vi "Dashboard Main.vi"() -> ()   [LabVIEW 2012]
uses:
  2012/code/Dashboard/High Priority Dash Data.ctl
  Control 3.ctl
  Control 4.ctl
  Control 2.ctl
  Control 5.ctl
  <vilib>/event_ctls.llb/eventvkey.ctl
  high priority dash data.vi
  low priority dash data.vi
  <vilib>/Utility/config.llb/Read Key (String).vi
  <vilib>/Utility/config.llb/Read Key (I32).vi
  <vilib>/Utility/config.llb/Write Key (String).vi
  <vilib>/Utility/config.llb/Write Key (I32).vi
  <vilib>/Utility/config.llb/NI_LVConfig.lvlib
panel:
  out "Battery Value":dbl(slide) scale=0.0..14.0 scale format="%#_2e"
  out "Battery":sgl(graph)
  in  "Camera Settings":T1={"Frate Rate"=30, "Compression"=30, "Size"=1} {"Frate Rate" scale=1.0..30.0; "Size" items=["640x480", "320x240", "160x120"]}
  out "Mode":T2(ring)=enum."Auto Disabled"
  out "Camera IP":string
  out "JS1 Z":dbl(slide) scale=-1.0..1.0 scale format="%#_2e"
  out "JS2 Z":dbl(slide) scale=-1.0..1.0 scale format="%#_2e"
  out "Joystick 1":cluster{"X":dbl, "Y":dbl}[](graph)
  out "Joystick 2":cluster{"X":dbl, "Y":dbl}[](graph)
  out "JS Buttons 1":T3
  out "JS Buttons 2":T3
  out "MotorSlide4":dbl(slide) scale=-1.0..1.0 scale format="%#_2e"
  out "MotorSlide3":dbl(slide) scale=-1.0..1.0 scale format="%#_2e"
  out "MotorSlide2":dbl(slide) scale=-1.0..1.0 scale format="%#_2e"
  in  "MotorName3":string="Front Left"
  in  "MotorName4":string="Front Right"
  in  "MotorName1":string="Rear Left"
  in  "MotorName2":string="Rear Right"
  out "MotorChart4":dbl(graph)
  out "MotorChart3":dbl(graph)
  out "MotorChart2":dbl(graph)
  out "MotorSlide1":dbl(slide) scale=-1.0..1.0 scale format="%#_2e"
  out "MotorChart1":dbl(graph)
  out "Robot IP":string
  in  "Dashboard Tab":enum32{"Operation", "Test", "Checklist"}(tab)
  out "XY Graph":cluster{"Y":dbl[], "Y":dbl[]}[](graph)
  in  "Slider":dbl(slide) scale=0.0..100.0 scale format="%#_3g"
  in  "On/Off":bool caption="Solenoid"
  in  "Test Name":u16(ring) items=["Select the test to run..."]
  in  "Test Tree":string(tree)
  in  "Motor":cluster{"Value":dbl, "Enable":bool} {"Value" scale=-1.0..1.0 scale format="%#_3g"}
  out "Progress":T4 {"Test Progress" scale=0.0..100.0}
  in  "Rev/Fwd":cluster{"Forward":bool, "Reverse":bool}
  in  "Ring":u16(ring) items=["Auto", "Fixed indoor", "Fixed outdoor 1", "Fixed outdoor 2", "Fixed fluorescent 1", "Fixed fluorescent 2", "Hold current"]
  in  "Listbox":i32(listbox)
  in  "Viewer":T5(tab)
  out "Mbps":dbl format="%#.1g"
  in  "Enable":bool
  in  "DB Camera Config":bool
  out "Mbps":bool
  out "fps":dbl format="%#.1g"
  out "Image Error Message":string="Timeout in Camera Communications"
  out "Camera Image":T6(plugin-control)
  out "Buttons 1":cluster{"1":bool, "2":bool, "3":bool}
  out "Kinect 1":cluster{"X":dbl, "Y":dbl, "Z":dbl} {"X" scale=1.0..-1.0; "Y" scale=1.0..-1.0; "Z" scale=1.0..-1.0}
  out "Buttons 2":cluster{"1":bool, "2":bool, "3":bool}
  out "Kinect 2":cluster{"X":dbl, "Y":dbl, "Z":dbl} {"X" scale=1.0..-1.0; "Y" scale=1.0..-1.0; "Z" scale=1.0..-1.0}
  out "Version":string
  out "Skeleton Picture":picture
  out "Players":i8
  out "Tree":string(tree)
  # "Drive & Motors"
  # "Robot IP:"
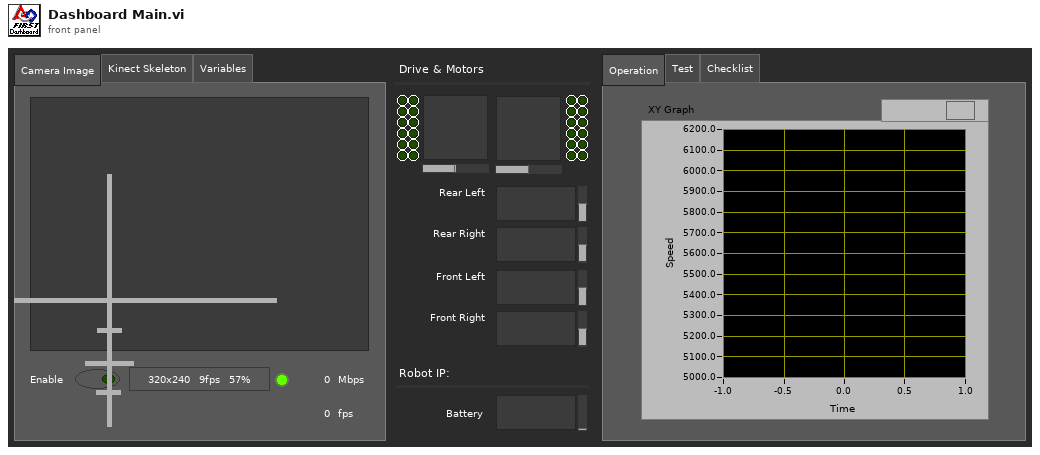
[diagram p1: front panel]
types:
  T1 = cluster{"Frate Rate":i32, "Compression":i32, "Size":u16}
  T2 = enum8{"Tele-Op Disabled", "Tele-Op Enabled", "Auto Disabled", "Auto Enabled", "Test Disabled", "Test Enabled", ""}
  T3 = cluster{bool, bool, bool, bool, bool, bool, bool, bool, bool, bool, bool, bool}
  T4 = cluster{"Test Progress":u8, "Test Progress Text":string}
  T5 = enum32{"Camera Image", "Kinect Skeleton", "Variables"}
  T6 = typedef "IMAQ Image.ctl" = refnum<image>
  T7 = typedef "Control 4.ctl" = cluster{"shooter speed":dbl}
  T8 = typedef "Control 3.ctl" = cluster{"shooter speed":dbl}
  T9 = typedef "High Priority Dash Data.ctl" = cluster{cluster{bool, i32, i32, i32, i32}, cluster{bool, i32, i32, i32, i32}, cluster{bool, i32, i32, i32, i32}, cluster{bool, i32, i32, i32, i32}}
  T10 = typedef "Image Type" = u32
  T11 = typedef "LVBoundsTypeDef.ctl" = cluster{"Width":u32, "Height":u32}
  T12 = typedef "SkeletonTrackState.ctl" = enum32{"NotTracked", "PositionOnly", "Tracked"}
  T13 = cluster{"TrackingState":u8[], "Position":cluster{"x":sgl, "y":sgl, "z":sgl}, cluster{"x":sgl, "y":sgl, "z":sgl, sgl}[], "TrackState":T12}
  T14 = cluster{cluster{"ScaledToPercentRange":dbl, "ScaledToPercentRange":dbl, "ScaledToPercentRange":dbl}, cluster{bool, bool, bool}}[]
  T15 = cluster{cluster{"ScaledToPercentRange":dbl, "ScaledToPercentRange":dbl, "ScaledToPercentRange":dbl}, cluster{bool, bool, bool}}
  T16 = cluster{"ScaledToPercentRange":dbl, "ScaledToPercentRange":dbl, "ScaledToPercentRange":dbl}
  T17 = typedef "LVRectTypeDef.ctl" = cluster{"Left":i16, "Top":i16, "Right":i16, "Bottom":i16}
  T18 = typedef "Control 5.ctl" = cluster{dbl}
  T19 = typedef "Control 2.ctl" = cluster{"shooter speed":dbl}
  T20 = cluster{"Competition mode":bool, "Robot Link":bool, "Autonomous":bool, "Enabled":bool, "E-Stop":bool, "Simulated":bool, "TestMode":bool, "Docked Window":bool}
  T21 = cluster{"Boolean Array[0]":bool, "Boolean Array[1]":bool, "Boolean Array[2]":bool, "Boolean Array[3]":bool, "Boolean Array[4]":bool, "Boolean Array[5]":bool, "Boolean Array[6]":bool, "Boolean Array[7]":bool, "Boolean Array[8]":bool, "Boolean Array[9]":bool, "Boolean Array[10]":bool, "Boolean Array[11]":bool}
  T22 = typedef "NI_LVConfig.lvlib/Config Data RefNum.ctl" = refnum<k1>
  T23 = typedef "eventvkey.ctl" = enum16{"ASCII", "Enter", "Return", "Shift", "Ctrl", "Alt", "Cmd", "Opt", "Caps", "NumLock", "Clear", "Break", "Up", "Down", "Left", "Right", "Insert", "Delete", "Home", "End", "PageUp", "PageDown", "Escape", "Help", "Pause", "ScrollLock", "F1", "F2", "F3", "F4", "F5", "F6", "F7", "F8", "F9", "F10", "F11", "F12", "F13", "F14", "F15", "F16", "F17", "F18", "F19", "F20", "F21", "F22", "F23", "F24", "Play", "VolumeUp", "VolumeDown", "Mute", "Two Byte Char"}
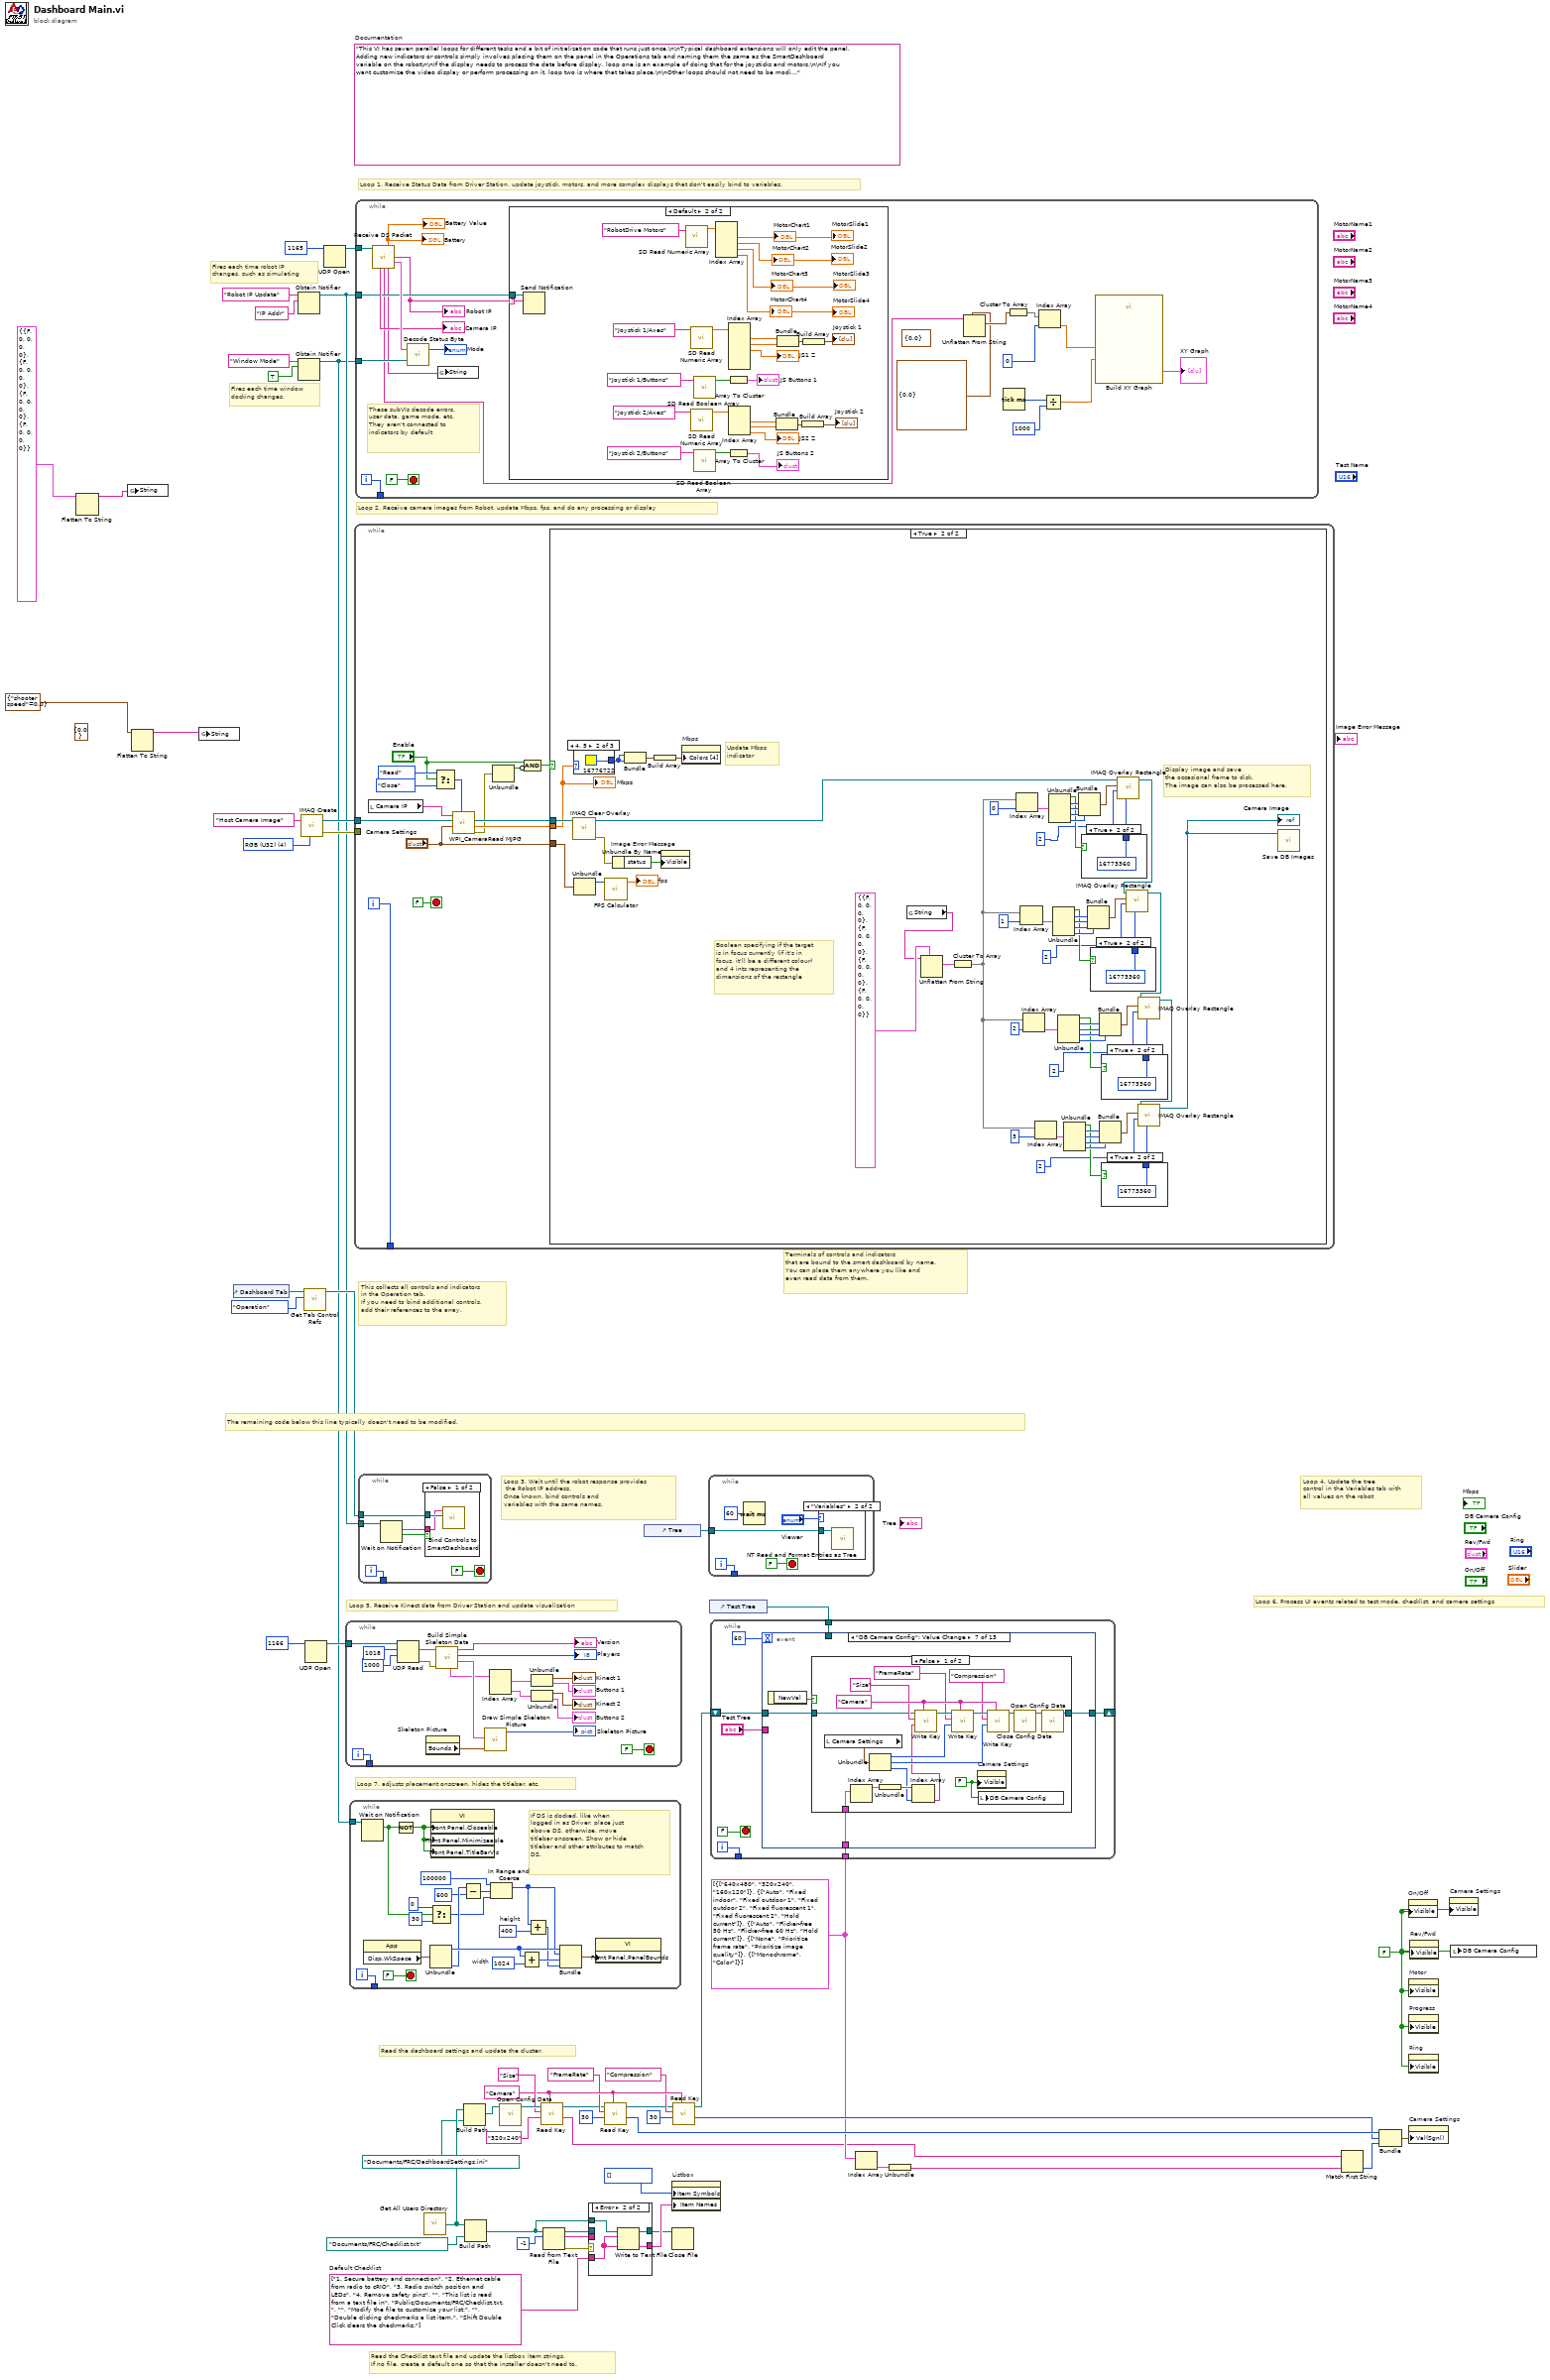
[diagram p0: block diagram]
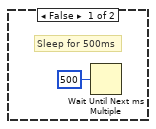
[diagram p3: hidden frame]
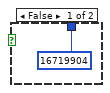
[diagram p4: hidden frame]
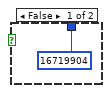
[diagram p5: hidden frame]
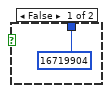
[diagram p6: hidden frame]
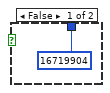
[diagram p7: hidden frame]
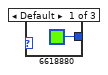
[diagram p8: hidden frame]
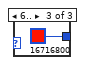
[diagram p9: hidden frame]
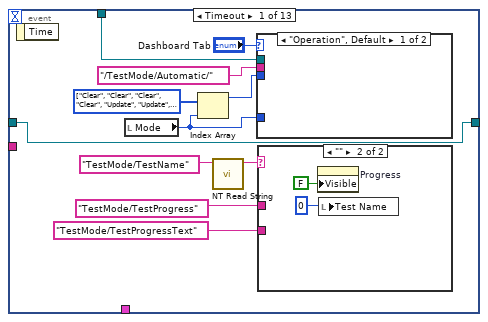
[diagram p11: hidden frame]
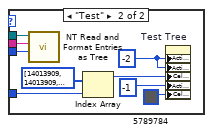
[diagram p12: hidden frame]
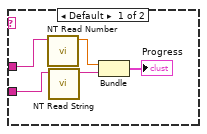
[diagram p13: hidden frame]
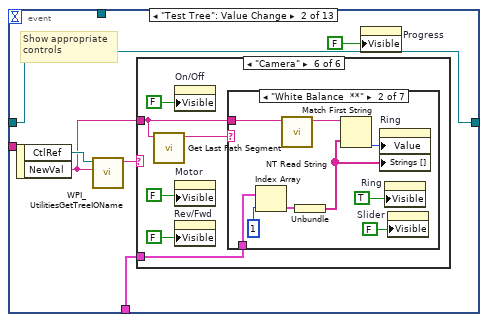
[diagram p14: hidden frame]
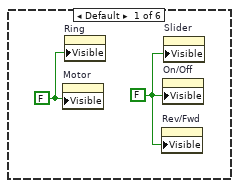
[diagram p15: hidden frame]
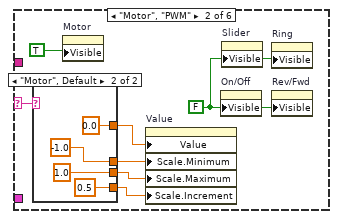
[diagram p16: hidden frame]
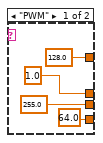
[diagram p17: hidden frame]
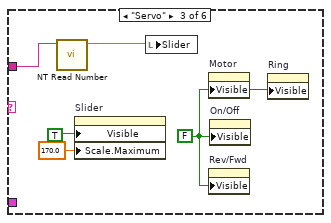
[diagram p18: hidden frame]
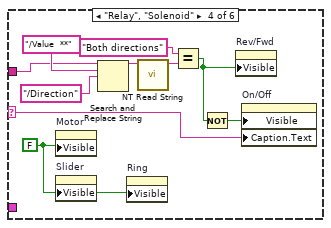
[diagram p19: hidden frame]
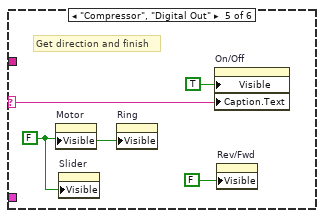
[diagram p20: hidden frame]
diagram:
  (unwired) T8 {"shooter speed"=0.0} ("Cluster")
  w25 = "Camera"
  w17 = cluster{string[]}[] [{["640x480", "320x240", "160x120"]}, {["Auto", "Fixed indoor", "Fixed outdoor 1", "Fixed outdoor 2", "Fixed fluorescent 1", "Fixed fluorescent 2", "Hold current"]}, {["Auto", "Flicker-free 50 Hz", "Flicker-free 60 Hz", "Hold current"]}, {["None", "Prioritize frame rate", "Prioritize image quality"]}, {["Monochrome", "Color"]}]
  w33 = string[] ["1. Secure battery and connection", "2. Ethernet cable from radio to cRIO", "3. Radio switch position and LEDs", "4. Remove safety pins", "", "This list is read from a text file in", "Public/Documents/FRC/Checklist.txt.", "", "Modify the file to customize your list.", "", "Double clicking checkmarks a list item.", "Shift Double Click clears the checkmarks."]  # Default Checklist
  w31 = FALSE ("Visible")
  (unwired) "This VI has seven parallel loops for different tasks and a bit of initialization code that runs just once.\n\nTypical dashboard extensions will only edit the panel. Adding new indicators or controls simply involves placing them on the panel in the Operations tab and naming them the same as the SmartDashboard variable on the robot\n\nIf the display needs to process the data before display, loop one is an example of doing that for the joysticks and motors.\n\nIf you want customize the video display or perform processing on it, loop two is where that takes place.\n\nOther loops should not need to be modified. They are pretty standard, and document the task they perform."  # Documentation
  w54 = T10 4 items=["Grayscale (U8)", "Grayscale (I16)", "Grayscale (SGL)", "Complex (CSG)", "RGB (U32)", "HSL (U32)", "RGB (U64)"] ("Image Type")
  # "Fires each time robot IP\nchanges, such as simulating"
  # "Fires each time window\ndocking changes."
  # "Read the Checklist text file and update the listbox item strings.\nIf no file, create a default one so that the installer doesn't need to."
  # "This collects all controls and indicators\nin the Operation tab.\nIf you need to bind additional controls,\nadd their references to the array."
  # "The remaining code below this line typically doesn't need to be modified."
  # "Loop 6. Process UI events related to test mode, checklist, and camera settings"
  # "Read the dashboard settings and update the cluster."
  # "Terminals of controls and indicators\nthat are bound to the smart dashboard by name.\nYou can place them anywhere you like and\neven read data from them."
  # "Loop 4. Update the tree\ncontrol in the Variables tab with\nall values on the robot"
  # "Loop 3. Wait until the robot response provides\n the Robot IP address.\nOnce known, bind controls and\nvariables with the same names."
  # "Loop 5. Receive Kinect data from Driver Station and update visualization"
  # "Loop 7. adjusts placement onscreen, hides the titlebar, etc."
  # "Loop 1. Receive Status Data from Driver Station, update joystick, motors, and more complex displays that don't easily bind to variables."
  # "Loop 2. Receive camera images from Robot, update Mbps, fps, and do any processing or display"
  n1 = Flatten To String(anything=T9 {{FALSE, 0, 0, 0, 0}, {FALSE, 0, 0, 0, 0}, {FALSE, 0, 0, 0, 0}, {FALSE, 0, 0, 0, 0}}) -> (data string=w3:string)  [unwired: 3 in, 2 out]
  n2 = global write "high priority dash data.vi" "String"(w3) -> ()
  n3 = Flatten To String(anything=T7 {"shooter speed"=0.0} ("Cluster")) -> (data string=w2:string)  [unwired: 3 in, 2 out]
  n4 = global write "low priority dash data.vi" "String"(w2) -> ()
  n5 = control-ref of="Dashboard Tab"() -> (w47:refnum<vi>)
  n6 = Obtain Notifier(name (unnamed)="Robot IP Update", notification data type="IP Addr" ("name (unnamed)")) -> (notifier out=w44:refnum<notifier>)  [unwired: 2 in, 2 out]
  n7 = Obtain Notifier(name (unnamed)="Window Mode", notification data type=TRUE) -> (notifier out=w37:refnum<notifier>)  [unwired: 2 in, 2 out]
  n8 = call "IMAQ Create"("Image Name"="Host Camera Image", "Image Type"=w54) -> ("New Image"=w52:T6, "error out"=w51:errorcluster)  [unwired: 2 in, 1 out]
  n9 = call <vilib>:"Get Tab Control Refs.vi"("Page Index"=enum32{"Operation", "Test"}."Operation" ("Dashboard Tab"), "TabControl in"=w47) -> ("ControlsOnPage"=w48:refnum<vi>[])  [unwired: 9 in]
  n10 = UDP Open(11:u16 1166 ("port")) -> (port=w49:refnum<k16>)  [unwired: 2 in, 4 out]
  n11 = UDP Open(11:u16 1165 ("port")) -> (port=w55:refnum<k16>)  [unwired: 2 in, 4 out]
  n12 = while {
    tunnel: w49 -> [w73]
    tunnel: [w58] -> _
    i -> [w58]
    stop <- FALSE stop-if-true
    n13 = UDP Read(connection ID=w73, max size (548)=1018 ("bytes to read"), timeout ms (25000)=1000) -> (data out=w67:string, error out=w57:errorcluster)  [unwired: 1 in, 3 out]
    n14 = property on="Skeleton Picture" class="Pict"() -> ("Bounds"=w69:T11)  [unwired: 2 in, 2 out]
    n15 = call "Build Simple Skeleton Data.vi"("error in (no error)"=w57, "data in"=w67) -> ("Skeleton Data"=w68:T13, "NumPlayers"=→"Players":i8, "Version String"=→"Version":string, "Simple Joystick Info"=w65:T14)  [unwired: 5 in, 1 out]
    n16 = call "Draw Simple Skeleton Picture.vi"("Bounds"=w69, "Simple Skeleton"=w68) -> ("new picture out"=→"Skeleton Picture":picture)  [unwired: 9 in]
    n17 = Index Array(array=w65) -> (element #1=w64:T15, element #2=w63:T15)  [unwired: 2 in]
    n18 = Unbundle(w64) -> (→"Kinect 1":T16, →"Buttons 1":cluster{bool, bool, bool})
    n19 = Unbundle(w63) -> (→"Kinect 2":T16, →"Buttons 2":cluster{bool, bool, bool})
  }
  n20 = while {
    tunnel: w37 -> [w94]
    tunnel: [w92] -> _
    i -> [w92]
    stop <- FALSE stop-if-true
    w84 = 1024  # width
    w87 = 400  # height
    # "If DS is docked, like when\nlogged in as Driver, place just\nabove DS, otherwise, move\ntitlebar onscreen. Show or hide\ntitlebar and other attributes to match\nDS."
    n21 = Wait on Notification(notifier=w94) -> (notification=w79:bool)  [unwired: 3 in, 3 out]
    n22 = property class="App"() -> ("Disp.WkSpace"=w90:T17)  [unwired: 2 in, 2 out]
    n23 = Not(x=w79) -> (.not. x?=w93:bool)
    n24 = Unbundle(w90) -> ("Left"=w88:i16, "Bottom"=w85:i16)  [unwired: 2 out]
    n25 = Select(t=0, s=w79, f=30) -> (s? t:f=w78:i32)
    n26 = property class="VI"("Front Panel.Closeable"=w93, "Front Panel.Minimizeable"=w93, "Front Panel.TitleBarVis"=w93) -> ()  [unwired: 2 in, 2 out]
    n27 = Subtract(x=w85, y=600) -> (x-y=w82:i32)
    n28 = In Range and Coerce(upper limit=100000, x=w82, lower limit=w78) -> (coerced(x)=w76:i32)  [unwired: 1 out]
    n29 = Add(x=w88, y=w84) -> (x+y=w89:i32)
    n30 = Add(x=w76, y=w87) -> (x+y=w86:i32)
    n31 = Bundle("Left"=w88, w76, w89, w86) -> (w91:cluster{"Left":i16, i32, i32, i32})  [unwired: 1 out]
    n32 = property class="VI"("Front Panel.PanelBounds"=w91) -> ()  [unwired: 2 in, 2 out]
  }
  n33 = while {
    tunnel: w52 -> [w105]
    tunnel: w51 -> [_]
    tunnel: [w108] -> _
    i -> [w108]
    stop <- FALSE stop-if-true
    n34 = local read "Camera IP"() -> (w107:string)
    n35 = Select(t=enum16{"Read", "Reopen", "Close"}."Read" ("Operation"), s="Enable", f=enum16{"Read", "Reopen", "Close"}."Close" ("Operation")) -> (s? t:f=w100:enum16{"Read", "Reopen", "Close"})
    n36 = call <vilib>:"WPI_CameraRead MJPG.vi"("Operation"=w100, "Camera Settings"="Camera Settings", "Image"=w105, "address"=w107) -> ("error out"=w99:errorcluster, "Bandwidth (kbps)"=w103:dbl, "Image Out"=w104:T6)  [unwired: 5 in]
    n37 = Unbundle(w99) -> ("status"=w97:bool)  [unwired: 2 out]
    n38 = Compound Arithmetic op=AND("Enable", invert w97) -> (w96:bool)
    n39 = case shown="True" w96 {
      tunnel: "Camera Settings" -> [_ w161]
      tunnel: w104 -> [_ w164]
      tunnel: w103 -> [_ w163]
      frame False {
        # "Sleep for 500ms"
        n40 = Wait Until Next ms Multiple(millisecond multiple=u32 500) -> ()  [unwired: 1 out]
      }
      frame True {
        # "Boolean specifying if the target\nis in focus currently (if it's in \nfocus, it'll be a different colour)\nand 4 ints representing the\ndimensions of the rectangle"
        # "Display image and save\nthe occasional frame to disk.\nThe image can also be processed here."
        # "Update Mbps\nindicator"
        n41 = call "IMAQ Clear Overlay"("Image"=w164) -> ("error out"=w168:errorcluster, "Image Out"=w113:T6)  [unwired: 2 in, 7 out]
        n42 = case shown="4, 5" w163 {
          tunnel: [u32 6618880 ("Color Box") u32 16776722 ("Color Box") u32 16716800 ("Color Box")] -> w165
          frame Default {
          }
          frame 4, 5 {
          }
          frame 6.. {
          }
        }
        n43 = Unbundle(w161) -> ("Frate Rate"=w160:i32)  [unwired: 2 out]
        n44 = call "FPS Calculator.vi"("Average Count"=w160) -> ("fps"=→"fps":dbl)  [unwired: 10 in]
        n45 = Unbundle By Name(w168) -> ("status"=w169:bool)
        n46 = Bundle("Color Box"=w165, "Color Box"=w165) -> (w167:cluster{"Color Box":u32, "Color Box":u32})  [unwired: 1 out]
        n47 = Build Array(w167) -> (w166:cluster{"Color Box":u32, "Color Box":u32}[])
        n48 = property on="Image Error Message" class="Str"("Visible"=w169) -> ()  [unwired: 2 in, 2 out]
        n49 = property on="Mbps" class="Bool (strict)"("Colors [4]"=w166) -> ()  [unwired: 2 in, 2 out]
        n50 = global read "high priority dash data.vi" "String"() -> (w114:string)
        n51 = Unflatten From String(type=T9 {{FALSE, 0, 0, 0, 0}, {FALSE, 0, 0, 0, 0}, {FALSE, 0, 0, 0, 0}, {FALSE, 0, 0, 0, 0}}, binary string=w114) -> (value=w151:T9)  [unwired: 1 in, 4 out]
        n52 = Cluster To Array(cluster=w151) -> (array=w111:cluster{bool, i32, i32, i32, i32}[])
        n53 = Index Array(array=w111, index=0) -> (element=w149:cluster{bool, i32, i32, i32, i32})
        n54 = Index Array(array=w111, index=1) -> (element=w140:cluster{bool, i32, i32, i32, i32})
        n55 = Index Array(array=w111, index=2) -> (element=w131:cluster{bool, i32, i32, i32, i32})
        n56 = Index Array(array=w111, index=3) -> (element=w122:cluster{bool, i32, i32, i32, i32})
        n57 = Unbundle(w149) -> (w152:bool, w153:i32, w154:i32, w156:i32, w155:i32)
        n58 = Unbundle(w140) -> (w142:bool, w143:i32, w144:i32, w146:i32, w145:i32)
        n59 = Unbundle(w131) -> (w133:bool, w134:i32, w135:i32, w137:i32, w136:i32)
        n60 = Unbundle(w122) -> (w124:bool, w125:i32, w126:i32, w128:i32, w127:i32)
        n61 = Bundle(w153, w154, w156, w155) -> (w158:cluster{i32, i32, i32, i32})  [unwired: 1 in]
        n62 = case shown="True" w152 {
          tunnel: [16719904 16773360] -> w157
          frame False {
          }
          frame True {
          }
        }
        n63 = Bundle(w143, w144, w146, w145) -> (w148:cluster{i32, i32, i32, i32})  [unwired: 1 in]
        n64 = case shown="True" w142 {
          tunnel: [16719904 16773360] -> w147
          frame False {
          }
          frame True {
          }
        }
        n65 = Bundle(w134, w135, w137, w136) -> (w139:cluster{i32, i32, i32, i32})  [unwired: 1 in]
        n66 = Bundle(w125, w126, w128, w127) -> (w130:cluster{i32, i32, i32, i32})  [unwired: 1 in]
        n67 = case shown="True" w133 {
          tunnel: [16719904 16773360] -> w138
          frame False {
          }
          frame True {
          }
        }
        n68 = case shown="True" w124 {
          tunnel: [16719904 16773360] -> w129
          frame False {
          }
          frame True {
          }
        }
        n69 = call "IMAQ Overlay Rectangle"("Color"=w157, "Drawing Mode (Frame)"=2, "Rectangle"=w158, "Image"=w113) -> ("Image Out"=w121:T6)  [unwired: 6 in, 1 out]
        n70 = call "IMAQ Overlay Rectangle"("Color"=w147, "Drawing Mode (Frame)"=2, "Rectangle"=w148, "Image"=w121) -> ("Image Out"=w120:T6)  [unwired: 6 in, 1 out]
        n71 = call "IMAQ Overlay Rectangle"("Color"=w138, "Drawing Mode (Frame)"=2, "Rectangle"=w139, "Image"=w120) -> ("Image Out"=w119:T6)  [unwired: 6 in, 1 out]
        n72 = call "IMAQ Overlay Rectangle"("Color"=w129, "Drawing Mode (Frame)"=2, "Rectangle"=w130, "Image"=w119) -> ("Image Out"=w112:T6)  [unwired: 6 in, 1 out]
        "Camera Image" <- w112
        n73 = call "Save DB Images.vi"("Image"=w112) -> ()  [unwired: 2 in, 1 out]
        "Mbps" <- w163
      }
    }
  }
  n74 = while {
    tunnel: w55 -> [w199]
    tunnel: w44 -> [w193]
    tunnel: w37 -> [w197]
    tunnel: [w194] -> _
    i -> [w194]
    stop <- FALSE stop-if-true
    (unwired) T19 {"shooter speed"=0.0} ("Cluster")
    # "These subVIs decode errors, user data, game mode, etc.\nThey aren't connected to indicators by default"
    n75 = call "Receive DS Packet.vi"("Recv Socket"=w199) -> ("Battery"=→"Battery" →"Battery Value":sgl, "Robot IP Address"=w192:string, "Status"=w200:T20, "Camera IP Address"=→"Camera IP":string, "Low Priority User Data"=w181:string, "High Priority User Data"=w191:string)  [unwired: 1 in, 8 out]
    "Robot IP" <- w192
    n76 = call "Decode Status Byte.vi"("Window Mode Notifier"=w197, "Status"=w200) -> ("Mode"=→"Mode":T2)  [unwired: 1 out]
    n77 = global write "high priority dash data.vi" "String"(w191) -> ()
    n78 = case shown="Default" w192 {
      selector: w192 -> [_ w202]
      tunnel: w193 -> [_ w203]
      frame "0.0.0.0" {
        # "Robot not responding, don't poll the variables"
      }
      frame Default {
        n79 = Send Notification(notification=w202, notifier=w203) -> ()  [unwired: 1 in, 2 out]
        n80 = call <vilib>:"SD Read Numeric Array.vi"("Name"="RobotDrive Motors") -> ("Numeric Array"=w226:dbl[])  [unwired: 8 in, 2 out]
        n81 = call <vilib>:"SD Read Numeric Array.vi"("Name"="Joystick 1/Axes") -> ("Numeric Array"=w219:dbl[])  [unwired: 8 in, 2 out]
        n82 = call <vilib>:"SD Read Numeric Array.vi"("Name"="Joystick 2/Axes") -> ("Numeric Array"=w213:dbl[])  [unwired: 8 in, 2 out]
        n83 = call <vilib>:"SD Read Boolean Array.vi"("Name"="Joystick 1/Buttons") -> ("Boolean Array"=w221:bool[])  [unwired: 8 in, 2 out]
        n84 = call <vilib>:"SD Read Boolean Array.vi"("Name"="Joystick 2/Buttons") -> ("Boolean Array"=w212:bool[])  [unwired: 8 in, 2 out]
        n85 = Index Array(array=w226) -> (element #1=→"MotorChart1" →"MotorSlide1":dbl, element #2=→"MotorSlide2" →"MotorChart2":dbl, element #3=→"MotorChart3" →"MotorSlide3":dbl, element #4=→"MotorChart4" →"MotorSlide4":dbl)  [unwired: 4 in]
        n86 = Array To Cluster(array=w221) -> (cluster=→"JS Buttons 1":T21)
        n87 = Array To Cluster(array=w212) -> (cluster=→"JS Buttons 2":T21)
        n88 = Index Array(array=w219) -> (element #1=w216:dbl, element #2=w217:dbl, element #3=→"JS1 Z":dbl)  [unwired: 6 in, 3 out]
        n89 = Index Array(array=w213) -> (element #1=w208:dbl, element #2=w207:dbl, element #3=→"JS2 Z":dbl)  [unwired: 3 in]
        n90 = Bundle("Numeric"=w208, "Numeric"=w207) -> (w209:cluster{"Numeric":dbl, "Numeric":dbl})  [unwired: 1 in]
        n91 = Bundle("Numeric"=w216, "Numeric"=w217) -> (w215:cluster{"Numeric":dbl, "Numeric":dbl})  [unwired: 1 in]
        n92 = Build Array(w209) -> (→"Joystick 2":cluster{"Numeric":dbl, "Numeric":dbl}[])
        n93 = Build Array(w215) -> (→"Joystick 1":cluster{"Numeric":dbl, "Numeric":dbl}[])
      }
    }
    n94 = Unflatten From String(type=T18 {0.0}, binary string=w181) -> (value=w189:T18)  [unwired: 1 in, 4 out]
    n95 = Tick Count (ms)() -> (millisecond timer value=w184:u32)
    n96 = Cluster To Array(cluster=w189) -> (array=w188:dbl[])
    n97 = Index Array(array=w188, index=0) -> (element=w186:dbl)
    n98 = Divide(x=w184, y=1000) -> (x/y=w183:dbl)
    n99 = call "Build XY Graph"("Y Input"=w183, "X Input"=w186) -> ("XY Graph"=→"XY Graph":cluster{"Y":dbl[], "Y":dbl[]}[])  [unwired: 3 in, 6 out]
  }
  n100 = while {
    tunnel: w48 -> [w235]
    tunnel: w44 -> [w232]
    tunnel: [w230] -> _
    i -> [w230]
    stop <- FALSE stop-if-true
    n101 = Wait on Notification(notifier=w232) -> (notification=w231:string, timed out?=w233:bool)  [unwired: 3 in, 2 out]
    n102 = case shown="False" w233 {
      tunnel: w235 -> [w237 _]
      tunnel: w231 -> [w236 _]
      frame False {
        n103 = call <vilib>:"Bind Controls to SmartDashboard.vi"("Bound Control Refs"=w237, "Server IP Address"=w236) -> ()  [unwired: 10 in]
      }
      frame True {
      }
    }
  }
  n104 = call "Get All Users Directory.vi"() -> ("All User Path"=w30:path)
  n105 = Build Path(base path=w30, name or relative path=path "Documents/FRC/DashboardSettings.ini") -> (appended path=w29:path)
  n106 = Build Path(base path=w30, name or relative path=path "Documents/FRC/Checklist.txt") -> (appended path=w34:path)
  n107 = call <vilib>:"Open Config Data.vi"("configuration file path"=w29) -> ("refnum"=w28:T22)  [unwired: 8 in, 2 out]
  n108 = call-poly <vilib>:"Read Key.vi"("section"=w25, "default value"="320x240", "key"="Size", "refnum"=w28) -> ("value"=w15:string, "refnum out"=w10:T22)  [unwired: 2 in, 4 out]
  n109 = Read from Text File(file (use dialog)=w34, count=-1 ("timeout ms (25000)")) -> (refnum out=w12:refnum<file>, text=w35:string[], error out=w36:errorcluster)  [unwired: 2 in, 1 out]
  n110 = case shown="Error" w36 {
    tunnel: w35 -> [w239 _]
    tunnel: [w239 w241] -> w32
    tunnel: w33 -> [_ w241]
    tunnel: w34 -> [_ w242]
    tunnel: [w238 w240] -> w11
    tunnel: w12 -> [w238 _]
    frame No Error {
    }
    frame Error {
      n111 = Write to Text File(file (use dialog)=w242, text=w241) -> (refnum out=w240:refnum<file>)  [unwired: 2 in, 2 out]
    }
  }
  n112 = call-poly <vilib>:"Read Key.vi"("section"=w25, "default value"=30, "key"="FrameRate", "refnum"=w10) -> ("value"=w20:i32, "refnum out"=w9:T22)  [unwired: 1 in, 5 out]
  n113 = control-ref of="Tree"() -> (w6:refnum<vi>)
  n114 = property on="Listbox" class="LstBox (strict)"("Item Symbols"=i32[] [], "Item Names"=w32) -> ()  [unwired: 2 in, 2 out]
  n115 = Close File(refnum=w11) -> ()  [unwired: 1 in, 2 out]
  n116 = call-poly <vilib>:"Read Key.vi"("section"=w25, "default value"=30, "key"="Compression", "refnum"=w9) -> ("value"=w19:i32, "refnum out"=w7:T22)  [unwired: 1 in, 5 out]
  n117 = while {
    tunnel: [w244] -> _
    tunnel: w6 -> [w243]
    i -> [w244]
    stop <- FALSE stop-if-true
    n118 = Wait (ms)(milliseconds to wait=u32 60) -> ()  [unwired: 1 out]
    n119 = case shown="\"Variables\"" "Viewer" {
      tunnel: w243 -> [_ w248]
      frame Default {
      }
      frame "Variables" {
        n120 = call <vilib>:"NT Read and Format Entries as Tree.vi"("Tree Refnum"=w248) -> ()  [unwired: 9 in, 2 out]
      }
    }
  }
  n121 = control-ref of="Test Tree"() -> (w5:refnum<vi>)
  n122 = while {
    tunnel: w17 -> [w253]
    shift-right: [w252] -> _
    shift-left: w7 -> [w251]
    tunnel: [w250] -> _
    tunnel: w5 -> [w249]
    i -> [w250]
    stop <- FALSE stop-if-true
    n123 = event shown="[6] \"DB Camera Config\": Value Change" {
      selector: _ -> [_ _ _ _ _ _ _ _ _ _ _ _ _]
      dyn-events: _ -> [_ _ _ _ _ _ _ _ _ _ _ _ _]
      timeout: u32 60 ("milliseconds to wait") -> [_ _ _ _ _ _ _ _ _ _ _ _ _]
      tunnel: w249 -> [w263 _ _ _ _ _ _ _ _ _ _ _ _]
      tunnel: "Test Tree" -> [_ _ _ _ _ _ _ _ w457 w465 w467 w471 w479]
      tunnel: w253 -> [_ w285 _ _ _ _ w421 w451 _ _ _ _ _]
      tunnel: [w257 w284 _ w387 w395 w407 w420 w444 w456 w463 w466 w470 w478] -> w252
      tunnel: w251 -> [w257 w284 _ w387 w395 w407 w419 w444 w456 w463 w466 w470 w478]
      event Timeout {
        w262 = enum16{"Update", "Clear"}[] [enum."Clear", enum."Clear", enum."Clear", enum."Clear", enum."Update", enum."Update", enum."Clear"] items=["Update", "Clear"]
        n124 = event-data() -> ()  [unwired: 1 in, 1 out]
        n125 = local read "Mode"() -> (w260:T2)
        n126 = Index Array(array=w262, index=w260) -> (element=w261:enum16{"Update", "Clear"})
        n127 = call <vilib>:"NT Read String.vi"("Name"="TestMode/TestName") -> ("String"=w266:string)  [unwired: 9 in, 1 out]
        n128 = case shown="\"Operation\", Default" "Dashboard Tab" {
          tunnel: w263 -> [_ w276]
          tunnel: "/TestMode/Automatic/" ("Name Pattern") -> [_ w275]
          tunnel: w261 -> [_ w274]
          tunnel: w260 -> [_ w272]
          frame "Operation", Default {
          }
          frame "Test" {
            w271 = -2 ("Active Item:Row Number")
            n129 = call <vilib>:"NT Read and Format Entries as Tree.vi"("Operation"=w274, "Name Pattern"=w275, "Tree Refnum"=w276) -> ()  [unwired: 7 in, 2 out]
            n130 = Index Array(array=u32[] [14013909, 14013909, 14013909, 14013909, 14013909, 16777215, 14013909], index=w272) -> (element=w270:u32)
            n131 = property on="Test Tree" class="Tree (strict)"("Active Item Row Number"=w271, "ActiveColNum"=w271, "CellBG"=w270, "Active Item Row Number"=-1 ("Active Item:Row Number"), "CellBG"=u32 5789784 ("Color Box")) -> ()  [unwired: 2 in, 2 out]
          }
        }
        n132 = case shown="\"\"" w266 {
          tunnel: "TestMode/TestProgress" ("Name") -> [w278 _]
          tunnel: "TestMode/TestProgressText" ("Name") -> [w277 _]
          frame Default {
            n133 = call <vilib>:"NT Read Number.vi"("Name"=w278) -> ("Numeric"=w279:dbl)  [unwired: 9 in, 1 out]
            n134 = call <vilib>:"NT Read String.vi"("Name"=w277) -> ("String"=w280:string)  [unwired: 9 in, 1 out]
            n135 = Bundle("Numeric"=w279, "String"=w280) -> (→"Progress":cluster{"Numeric":dbl, "String":string})  [unwired: 1 in]
          }
          frame "" {
            n136 = property on="Progress" class="Clust (strict)"("Visible"=FALSE) -> ()  [unwired: 2 in, 2 out]
            n137 = local write "Test Name"(u16 0) -> ()
          }
        }
      }
      event "Test Tree": Value Change {
        # "Show appropriate\ncontrols"
        n138 = event-data() -> ("CtlRef"=w288:refnum<vi>, "NewVal"=w286:string)  [unwired: 1 in]
        n139 = call <vilib>:"WPI_UtilitiesGetTreeIOName.vi"("NewVal"=w286, "TreeControl in"=w288) -> ("I/O Name"=w289:string)  [unwired: 9 in]
        n140 = case shown="\"Camera\"" w289 {
          selector: w289 -> [_ w296 _ w314 w323 _]
          tunnel: w286 -> [_ _ w311 w313 _ w330]
          tunnel: w285 -> [_ _ _ _ _ w329]
          frame Default {
            w291 = FALSE ("Visible")
            w290 = FALSE ("Visible")
            n141 = property on="Motor" class="Clust (strict)"("Visible"=w290) -> ()  [unwired: 2 in, 2 out]
            n142 = property on="Ring" class="Ring (strict)"("Visible"=w290) -> ()  [unwired: 2 in, 2 out]
            n143 = property on="Rev/Fwd" class="Clust (strict)"("Visible"=w291) -> ()  [unwired: 2 in, 2 out]
            n144 = property on="On/Off" class="Bool (strict)"("Visible"=w291) -> ()  [unwired: 2 in, 2 out]
            n145 = property on="Slider" class="Slide (strict)"("Visible"=w291) -> ()  [unwired: 2 in, 2 out]
          }
          frame "Motor", "PWM" {
            w297 = FALSE ("Visible")
            n146 = case shown="\"Motor\", Default" w296 {
              tunnel: [1.0 ("Value") -1.0 ("Value")] -> w295
              tunnel: [255.0 ("Value") 1.0 ("Value")] -> w294
              tunnel: [128.0 ("Value") 0.0 ("Value")] -> w293
              tunnel: [64.0 ("Value") 0.5 ("Value")] -> w292
              frame "PWM" {
              }
              frame "Motor", Default {
              }
            }
            n147 = property on="Motor" class="Clust (strict)"("Visible"=TRUE) -> ()  [unwired: 2 in, 2 out]
            n148 = property on="Value" class="Slide (strict)"("Value"=w293, "Scale.Minimum"=w295, "Scale.Maximum"=w294, "Scale.Increment"=w292) -> ()  [unwired: 2 in, 2 out]
            n149 = property on="On/Off" class="Bool (strict)"("Visible"=w297) -> ()  [unwired: 2 in, 2 out]
            n150 = property on="Slider" class="Slide (strict)"("Visible"=w297) -> ()  [unwired: 2 in, 2 out]
            n151 = property on="Ring" class="Ring (strict)"("Visible"=w297) -> ()  [unwired: 2 in, 2 out]
            n152 = property on="Rev/Fwd" class="Clust (strict)"("Visible"=w297) -> ()  [unwired: 2 in, 2 out]
          }
          frame "Servo" {
            w309 = FALSE ("Visible")
            n153 = call <vilib>:"NT Read Number.vi"("Name"=w311) -> ("Numeric"=w310:dbl)  [unwired: 9 in, 1 out]
            n154 = property on="Slider" class="Slide (strict)"("Visible"=TRUE, "Scale.Maximum"=170.0 ("Scale.Range:Maximum")) -> ()  [unwired: 2 in, 2 out]
            n155 = local write "Slider"(w310) -> ()
            n156 = property on="Motor" class="Clust (strict)"("Visible"=w309) -> ()  [unwired: 2 in, 2 out]
            n157 = property on="Rev/Fwd" class="Clust (strict)"("Visible"=w309) -> ()  [unwired: 2 in, 2 out]
            n158 = property on="On/Off" class="Bool (strict)"("Visible"=w309) -> ()  [unwired: 2 in, 2 out]
            n159 = property on="Ring" class="Ring (strict)"("Visible"=w309) -> ()  [unwired: 2 in, 2 out]
          }
          frame "Relay", "Solenoid" {
            w312 = FALSE ("Visible")
            n160 = property on="Motor" class="Clust (strict)"("Visible"=w312) -> ()  [unwired: 2 in, 2 out]
            n161 = property on="Slider" class="Slide (strict)"("Visible"=w312) -> ()  [unwired: 2 in, 2 out]
            n162 = Search and Replace String(input string=w313, search string="/Value  **", replace string="/Direction") -> (result string=w319:string)  [unwired: 5 in, 3 out]
            n163 = property on="Ring" class="Ring (strict)"("Visible"=w312) -> ()  [unwired: 2 in, 2 out]
            n164 = call <vilib>:"NT Read String.vi"("Name"=w319) -> ("String"=w317:string)  [unwired: 9 in, 1 out]
            n165 = Equal?(x="Both directions", y=w317) -> (x = y?=w315:bool)
            n166 = Not(x=w315) -> (.not. x?=w316:bool)
            n167 = property on="Rev/Fwd" class="Clust (strict)"("Visible"=w315) -> ()  [unwired: 2 in, 2 out]
            n168 = property on="On/Off" class="Bool (strict)"("Visible"=w316, "Caption.Text"=w314) -> ()  [unwired: 2 in, 2 out]
          }
          frame "Compressor", "Digital Out" {
            w322 = FALSE ("Visible")
            # "Get direction and finish"
            n169 = property on="Motor" class="Clust (strict)"("Visible"=w322) -> ()  [unwired: 2 in, 2 out]
            n170 = property on="Slider" class="Slide (strict)"("Visible"=w322) -> ()  [unwired: 2 in, 2 out]
            n171 = property on="Ring" class="Ring (strict)"("Visible"=w322) -> ()  [unwired: 2 in, 2 out]
            n172 = property on="On/Off" class="Bool (strict)"("Visible"=TRUE, "Caption.Text"=w323) -> ()  [unwired: 2 in, 2 out]
            n173 = property on="Rev/Fwd" class="Clust (strict)"("Visible"=FALSE) -> ()  [unwired: 2 in, 2 out]
          }
          frame "Camera" {
            n174 = call <vilib>:"Get Last Path Segment.vi"("String in"=w330) -> ("String out"=w331:string)  [unwired: 10 in]
            n175 = property on="On/Off" class="Bool (strict)"("Visible"=FALSE) -> ()  [unwired: 2 in, 2 out]
            n176 = property on="Motor" class="Clust (strict)"("Visible"=FALSE) -> ()  [unwired: 2 in, 2 out]
            n177 = property on="Rev/Fwd" class="Clust (strict)"("Visible"=FALSE) -> ()  [unwired: 2 in, 2 out]
            n178 = case shown="\"White Balance  **\"" w331 {
              tunnel: w330 -> [w337 w346 w355 w364 w373 _ w379]
              tunnel: w329 -> [w335 w343 w352 w361 w370 _ _]
              frame "Size  **" {
                n179 = Index Array(array=w335) -> (element=w334:cluster{string[]})  [unwired: 1 in]
                n180 = call <vilib>:"NT Read String.vi"("Name"=w337) -> ("String"=w336:string)  [unwired: 9 in, 1 out]
                n181 = Unbundle(w334) -> (w332:string[])
                n182 = Match First String(2:w332, 3:w336) -> (0:w333:i32)  [unwired: 1 out]
                n183 = property on="Ring" class="Ring (strict)"("Value"=w333, "Strings []"=w332) -> ()  [unwired: 2 in, 2 out]
                n184 = property on="Ring" class="Ring (strict)"("Visible"=TRUE) -> ()  [unwired: 2 in, 2 out]
                n185 = property on="Slider" class="Slide (strict)"("Visible"=FALSE) -> ()  [unwired: 2 in, 2 out]
              }
              frame "White Balance  **" {
                n186 = Index Array(array=w343, index=1) -> (element=w344:cluster{string[]})
                n187 = call <vilib>:"NT Read String.vi"("Name"=w346) -> ("String"=w345:string)  [unwired: 9 in, 1 out]
                n188 = Unbundle(w344) -> (w341:string[])
                n189 = Match First String(2:w341, 3:w345) -> (0:w340:i32)  [unwired: 1 out]
                n190 = property on="Ring" class="Ring (strict)"("Value"=w340, "Strings []"=w341) -> ()  [unwired: 2 in, 2 out]
                n191 = property on="Ring" class="Ring (strict)"("Visible"=TRUE) -> ()  [unwired: 2 in, 2 out]
                n192 = property on="Slider" class="Slide (strict)"("Visible"=FALSE) -> ()  [unwired: 2 in, 2 out]
              }
              frame "Exposure  **" {
                n193 = Index Array(array=w352, index=2) -> (element=w353:cluster{string[]})
                n194 = call <vilib>:"NT Read String.vi"("Name"=w355) -> ("String"=w354:string)  [unwired: 9 in, 1 out]
                n195 = Unbundle(w353) -> (w349:string[])
                n196 = Match First String(2:w349, 3:w354) -> (0:w350:i32)  [unwired: 1 out]
                n197 = property on="Ring" class="Ring (strict)"("Value"=w350, "Strings []"=w349) -> ()  [unwired: 2 in, 2 out]
                n198 = property on="Ring" class="Ring (strict)"("Visible"=TRUE) -> ()  [unwired: 2 in, 2 out]
                n199 = property on="Slider" class="Slide (strict)"("Visible"=FALSE) -> ()  [unwired: 2 in, 2 out]
              }
              frame "Exposure Priority  **" {
                n200 = Index Array(array=w361, index=3) -> (element=w362:cluster{string[]})
                n201 = call <vilib>:"NT Read String.vi"("Name"=w364) -> ("String"=w363:string)  [unwired: 9 in, 1 out]
                n202 = Unbundle(w362) -> (w358:string[])
                n203 = Match First String(2:w358, 3:w363) -> (0:w359:i32)  [unwired: 1 out]
                n204 = property on="Ring" class="Ring (strict)"("Value"=w359, "Strings []"=w358) -> ()  [unwired: 2 in, 2 out]
                n205 = property on="Ring" class="Ring (strict)"("Visible"=TRUE) -> ()  [unwired: 2 in, 2 out]
                n206 = property on="Slider" class="Slide (strict)"("Visible"=FALSE) -> ()  [unwired: 2 in, 2 out]
              }
              frame "Color Enable  **" {
                n207 = Index Array(array=w370, index=4) -> (element=w371:cluster{string[]})
                n208 = call <vilib>:"NT Read String.vi"("Name"=w373) -> ("String"=w372:string)  [unwired: 9 in, 1 out]
                n209 = Unbundle(w371) -> (w367:string[])
                n210 = Match First String(2:w367, 3:w372) -> (0:w368:i32)  [unwired: 1 out]
                n211 = property on="Ring" class="Ring (strict)"("Value"=w368, "Strings []"=w367) -> ()  [unwired: 2 in, 2 out]
                n212 = property on="Ring" class="Ring (strict)"("Visible"=TRUE) -> ()  [unwired: 2 in, 2 out]
                n213 = property on="Slider" class="Slide (strict)"("Visible"=FALSE) -> ()  [unwired: 2 in, 2 out]
              }
              frame Default {
                n214 = property on="Ring" class="Ring (strict)"("Visible"=FALSE) -> ()  [unwired: 2 in, 2 out]
                n215 = property on="Slider" class="Slide (strict)"("Visible"=FALSE) -> ()  [unwired: 2 in, 2 out]
              }
              frame "Brightness  **", "Color Level  **", "Compression  **", "FPS  **", "Sharpness  **" {
                n216 = call <vilib>:"NT Read Number.vi"("Name"=w379) -> ("Numeric"=w378:dbl)  [unwired: 9 in, 1 out]
                n217 = local write "Slider"(w378) -> ()
                n218 = property on="Slider" class="Slide (strict)"("Visible"=TRUE, "Scale.Maximum"=100.0 ("Scale.Range:Maximum")) -> ()  [unwired: 2 in, 2 out]
                n219 = property on="Ring" class="Ring (strict)"("Visible"=FALSE) -> ()  [unwired: 2 in, 2 out]
              }
            }
          }
        }
        n220 = property on="Progress" class="Clust (strict)"("Visible"=FALSE) -> ()  [unwired: 2 in, 2 out]
      }
      event "Test Name": Mouse Enter {
        # "Populate the ring with the list of tests"
        n221 = event-data() -> ()  [unwired: 1 in, 1 out]
        n222 = call <vilib>:"NT Read String Array.vi"("Name"="TestMode/TestList") -> ("String Array"=w386:string[])  [unwired: 9 in, 1 out]
        n223 = Build Array (concatenate)("Select the test to run...", w386) -> (w385:string[])
        n224 = property on="Test Name" class="Ring (strict)"("Strings []"=w385) -> ()  [unwired: 2 in, 2 out]
      }
      event "Test Name": Value Change {
        w388 = FALSE ("Visible")
        # "Tell the robot the test name to run"
        n225 = event-data() -> ("NewVal"=w392:u16)  [unwired: 1 in]
        n226 = property on="Test Name" class="Ring (strict)"() -> ("Strings []"=w393:string[])  [unwired: 2 in, 2 out]
        n227 = local write "Progress"(T4 {"Test Progress"=0, "Test Progress Text"=""} ("Progress")) -> ()
        n228 = Index Array(array=w393, index=w392) -> (element=w391:string)
        n229 = call <vilib>:"NT Write String.vi"("String"=w391, "Name"="TestMode/TestName") -> ()  [unwired: 9 in, 1 out]
        n230 = property on="Progress" class="Clust (strict)"("Visible"=TRUE) -> ()  [unwired: 2 in, 2 out]
        n231 = property on="Motor" class="Clust (strict)"("Visible"=w388) -> ()  [unwired: 2 in, 2 out]
        n232 = property on="Slider" class="Slide (strict)"("Visible"=w388) -> ()  [unwired: 2 in, 2 out]
        n233 = property on="On/Off" class="Bool (strict)"("Visible"=w388) -> ()  [unwired: 2 in, 2 out]
        n234 = property on="Rev/Fwd" class="Clust (strict)"("Visible"=w388) -> ()  [unwired: 2 in, 2 out]
        n235 = property on="Ring" class="Ring (strict)"("Visible"=w388) -> ()  [unwired: 2 in, 2 out]
      }
      event "Listbox": Double Click {
        n236 = event-data() -> ("PlatMods.Shift"=w396:bool, "Row"=w398:i32)  [unwired: 1 in]
        n237 = case shown="False" w396 {
          tunnel: w398 -> [w402 _]
          tunnel: 1 -> [w401 _]
          frame False {
            n238 = property on="Listbox" class="LstBox (strict)"() -> ("Item Symbols"=w400:i32[])  [unwired: 2 in, 2 out]
            n239 = Replace Array Subset(array=w400, new element=w401, index=w402) -> (w399:i32[])
            n240 = property on="Listbox" class="LstBox (strict)"("Item Symbols"=w399) -> ()  [unwired: 2 in, 2 out]
          }
          frame True {
            w403 = 0 ("Top Row")
            n241 = property on="Listbox" class="LstBox (strict)"() -> ("Number of Rows"=w405:u32)  [unwired: 2 in, 2 out]
            n242 = Initialize Array(0, w405) -> (w404:i32[])
            n243 = property on="Listbox" class="LstBox (strict)"("Top Row"=w403, "Value"=w403, "Item Symbols"=w404) -> ()  [unwired: 2 in, 2 out]
          }
        }
      }
      event "Listbox": Key Down {
        n244 = event-data() -> ("VKey"=w409:T23)  [unwired: 1 in]
        n245 = case shown="\"Left\", \"Right\"" w409 {
          selector: w409 -> [w414 _]
          tunnel: eventvkey."Left" ("VKey") -> [w412 _]
          frame "Left", "Right" {
            n246 = Equal?(x=w412, y=w414) -> (x = y?=w413:bool)
            n247 = Select(t=0, s=w413, f=1) -> (s? t:f=w415:i32)
            n248 = property on="Listbox" class="LstBox (strict)"() -> ("Item Symbols"=w418:i32[])  [unwired: 2 in, 2 out]
            n249 = Replace Array Subset(array=w418, new element=w415, index="Listbox") -> (w417:i32[])
            n250 = property on="Listbox" class="LstBox (strict)"("Item Symbols"=w417) -> ()  [unwired: 2 in, 2 out]
          }
          frame Default {
          }
        }
      }
      event "DB Camera Config": Value Change {
        n251 = event-data() -> ("NewVal"=w422:bool)  [unwired: 1 in]
        n252 = case shown="False" w422 {
          tunnel: w421 -> [w431 _]
          tunnel: [w424 w442] -> w420
          tunnel: w419 -> [w423 w442]
          frame False {
            w438 = "Camera"
            w441 = FALSE ("Visible")
            n253 = local read "Camera Settings"() -> (w430:T1)
            n254 = Index Array(array=w431) -> (element=w434:cluster{string[]})  [unwired: 1 in]
            n255 = Unbundle(w430) -> ("Frate Rate"=w429:i32, "Compression"=w428:i32, "Size"=w432:u16)
            n256 = Unbundle(w434) -> (w433:string[])
            n257 = Index Array(array=w433, index=w432) -> (element=w427:string)
            n258 = call-poly <vilib>:"Write Key.vi"("section"=w438, "value"=w427, "key"="Size", "refnum"=w423) -> ("refnum out"=w440:T22)  [unwired: 2 in, 5 out]
            n259 = call-poly <vilib>:"Write Key.vi"("section"=w438, "value"=w429, "key"="FrameRate", "refnum"=w440) -> ("refnum out"=w439:T22)  [unwired: 1 in, 6 out]
            n260 = property on="Camera Settings" class="Clust (strict)"("Visible"=w441) -> ()  [unwired: 2 in, 2 out]
            n261 = local write "DB Camera Config"(w441) -> ()
            n262 = call-poly <vilib>:"Write Key.vi"("section"=w438, "value"=w428, "key"="Compression", "refnum"=w439) -> ("refnum out"=w425:T22)  [unwired: 1 in, 6 out]
            n263 = call <vilib>:"Close Config Data.vi"("refnum"=w425) -> ("file path"=w426:path)  [unwired: 2 in, 8 out]
            n264 = call <vilib>:"Open Config Data.vi"("configuration file path"=w426) -> ("refnum"=w424:T22)  [unwired: 8 in, 2 out]
          }
          frame True {
            n265 = property on="Camera Settings" class="Clust (strict)"("Visible"=TRUE) -> ()  [unwired: 2 in, 2 out]
          }
        }
      }
      event "Camera Settings": Value Change {
        n266 = event-data() -> ("NewVal"=w455:T1)  [unwired: 1 in]
        n267 = Index Array(array=w451) -> (element=w450:cluster{string[]})  [unwired: 1 in]
        n268 = Unbundle(w455) -> ("Frate Rate"=w446:i32, "Compression"=w445:i32, "Size"=w448:u16)
        n269 = Unbundle(w450) -> (w449:string[])
        n270 = Index Array(array=w449, index=w448) -> (element=w447:string)
        n271 = Format Into String(format string="%s   %dfps   %d%%", w447, w446, w445) -> (resulting string=w452:string)  [unwired: 2 in, 1 out]
        n272 = Build Array(w452) -> (w453:string[])
        n273 = property on="DB Camera Config" class="Bool (strict)"("Strings [4]"=w453) -> ()  [unwired: 2 in, 2 out]
      }
      event "Motor.Enable": Value Change {
        n274 = event-data() -> ("NewVal"=w461:bool)  [unwired: 1 in]
        n275 = Unbundle("Motor") -> ("Value"=w460:dbl)  [unwired: 1 out]
        n276 = Select(t=w460, s=w461, f=0.0) -> (s? t:f=w458:dbl)
        n277 = call <vilib>:"NT Write Number.vi"("Numeric"=w458, "Name"=w457) -> ()  [unwired: 9 in, 1 out]
      }
      event "Slider": Value Change {
        n278 = event-data() -> ("NewVal"=w464:dbl)  [unwired: 1 in]
        n279 = call <vilib>:"NT Write Number.vi"("Numeric"=w464, "Name"=w465) -> ()  [unwired: 9 in, 1 out]
      }
      event "On/Off": Value Change {
        n280 = event-data() -> ("NewVal"=w469:bool)  [unwired: 1 in]
        n281 = Boolean To (0,1)(Boolean=w469) -> (0, 1=w468:i16)
        n282 = call <vilib>:"NT Write Number.vi"("Numeric"=w468, "Name"=w467) -> ()  [unwired: 9 in, 1 out]
      }
      event "Rev/Fwd": Value Change {
        n283 = event-data() -> ("NewVal.Forward"=w477:bool, "NewVal.Reverse"=w476:bool)  [unwired: 1 in]
        n284 = Boolean To (0,1)(Boolean=w477) -> (0, 1=w473:i16)
        n285 = Boolean To (0,1)(Boolean=w476) -> (0, 1=w475:i16)
        n286 = Negate(x=w475) -> (-x=w474:i16)
        n287 = Add(x=w473, y=w474) -> (x+y=w472:i16)
        n288 = call <vilib>:"NT Write Number.vi"("Numeric"=w472, "Name"=w471) -> ()  [unwired: 9 in, 1 out]
      }
      event "Ring": Value Change {
        n289 = event-data() -> ("NewVal"=w481:u16)  [unwired: 1 in]
        n290 = property on="Ring" class="Ring (strict)"() -> ("Strings []"=w482:string[])  [unwired: 2 in, 2 out]
        n291 = Index Array(array=w482, index=w481) -> (element=w480:string)
        n292 = call <vilib>:"NT Write String.vi"("String"=w480, "Name"=w479) -> ()  [unwired: 9 in, 1 out]
      }
    }
  }
  n293 = Index Array(array=w17) -> (element=w18:cluster{string[]})  [unwired: 1 in]
  n294 = Unbundle(w18) -> (w16:string[])
  n295 = Match First String(2:w16, 3:w15) -> (0:w14:i32)  [unwired: 1 out]
  n296 = Bundle("value"=w20, "value"=w19, "index"=w14) -> (w8:cluster{"value":i32, "value":i32, "index":i32})  [unwired: 1 out]
  n297 = property on="On/Off" class="Bool (strict)"("Visible"=w31) -> ()  [unwired: 2 in, 2 out]
  n298 = property on="Motor" class="Clust (strict)"("Visible"=w31) -> ()  [unwired: 2 in, 2 out]
  n299 = property on="Progress" class="Clust (strict)"("Visible"=w31) -> ()  [unwired: 2 in, 2 out]
  n300 = property on="Ring" class="Ring (strict)"("Visible"=w31) -> ()  [unwired: 2 in, 2 out]
  n301 = property on="Camera Settings" class="Clust (strict)"("Val(Sgnl)"=w8) -> ()  [unwired: 2 in, 2 out]
  n302 = property on="Rev/Fwd" class="Clust (strict)"("Visible"=w31) -> ()  [unwired: 2 in, 2 out]
  n303 = property on="Camera Settings" class="Clust (strict)"("Visible"=w31) -> ()  [unwired: 2 in, 2 out]
  n304 = local write "DB Camera Config"(w31) -> ()
